vi "Reference To Calling VI.vi"(2 "error in":errorcluster, 3 "Call Level (2)":i32=2) -> (0 "error out":errorcluster, 1 "VI Reference":refnum<vi>)   [LabVIEW 2010]
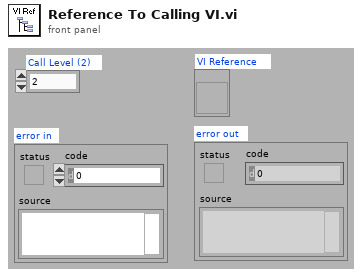
[diagram p1: front panel]
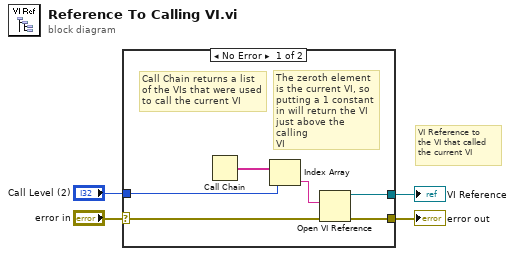
[diagram p0: block diagram]
diagram:
  # "VI Reference to \nthe VI that called\nthe current VI"
  n1 = case shown="No Error" "error in" {
    selector: "error in" -> [w5 w11]
    tunnel: "Call Level (2)" -> [w9 _]
    tunnel: [w7 _] -> w3
    tunnel: [w6 w11] -> w2
    frame No Error {
      # "The zeroth element\nis the current VI, so\nputting a 1 constant\nin will return the VI \njust above the calling\nVI"
      # "Call Chain returns a list\nof the VIs that were used\nto call the current VI"
      n2 = Call Chain() -> (call chain=w10:string[])
      n3 = Index Array(array=w10, index=w9) -> (element=w8:string)
      n4 = Open VI Reference(vi path=w8, error in (no error)=w5) -> (vi reference=w7:refnum<vi>, error out=w6:errorcluster)  [unwired: 4 in]
    }
    frame Error {
    }
  }
  "VI Reference" <- w3
  "error out" <- w2
